vi "Units to Display Units.vi"(10 "Units":string) -> (2 "Display units":string)   [LabVIEW 2021]
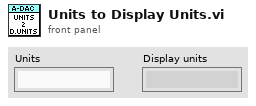
[diagram p1: front panel]
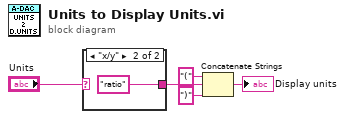
[diagram p0: block diagram]
diagram:
  n1 = case shown="\"x/y\"" "Units" {
    selector: "Units" -> [w6 _]
    tunnel: [w6 "ratio"] -> w3
    frame Default {
    }
    frame "x/y" {
    }
  }
  n2 = Concatenate Strings("(" ("string"), w3, ")" ("string")) -> (→"Display units":string)
